vi "Linear Fit (single).vi"(8 "error in (no error)":errorcluster, 9 "Type":enum16{"y vs x", "x vs y"}(ring), 11 "XY-data":cluster{"X-array":dbl[], "Y-array":dbl[]}) -> (0 "error out":errorcluster, 2 "Best Fit":cluster{"X-array":dbl[], "Y-array":dbl[]} {"Y-array" format="%.2p"; "X-array" format="%.2p"}, 3 "XY-data out":cluster{"X-array":dbl[], "Y-array":dbl[]}, 4 "slope":dbl, 5 "Lower Bound":cluster{"X-array":dbl[], "Y-array":dbl[]}, 6 "intercept":dbl, 7 "Upper Bound":cluster{"X-array":dbl[], "Y-array":dbl[]})   [LabVIEW 2019, in "xy_utilities.lvlib"]
doc: "Performs a linear fit using linear LS algorithm.\n\nWire data to the data input to determine the polymorphic instance to use or manually select the instance."
uses:
  xy_utilities.lvlib
  <vilib>/Analysis/6fits.llb/Curve Fitting Criteria.ctl
  Swap X and Y (single).vi
  <vilib>/Analysis/6fits.llb/Confidence Interval (Linear).vi
  <vilib>/Analysis/NI_AALPro.lvlib
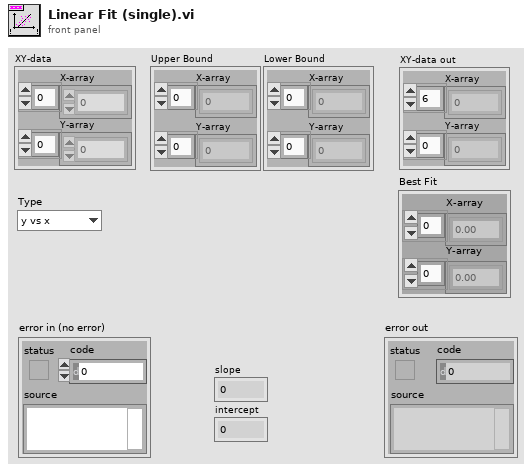
[diagram p1: front panel]
types:
  T1 = typedef "NI_AALPro.lvlib/Curve Fitting Criteria.ctl" = u16
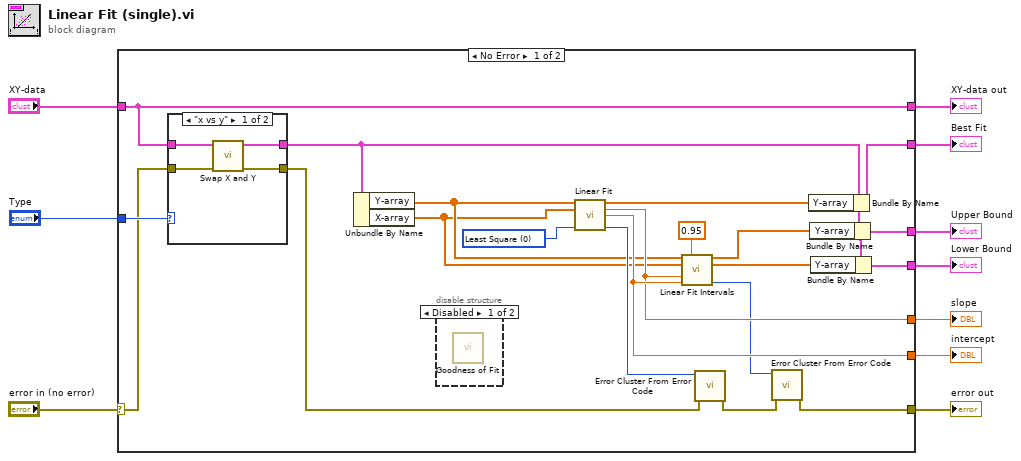
[diagram p0: block diagram]
diagram:
  n1 = case shown="No Error" "error in (no error)" {
    selector: "error in (no error)" -> [w30 w39]
    tunnel: [w18 w39] -> w9
    tunnel: "XY-data" -> [w28 w38]
    tunnel: [w29 _] -> w7
    tunnel: "Type" -> [w31 _]
    tunnel: [w28 w38] -> w5
    tunnel: [w22 _] -> w4
    tunnel: [w23 _] -> w3
    tunnel: [w12 _] -> w2
    tunnel: [w11 _] -> w1
    frame No Error {
      w24 = T1 0 items=["Least Square", "Least Absolute Residual", "Bisquare"] ("method")
      n2 = case shown="\"x vs y\"" w31 {
        tunnel: w28 -> [w35 w37]
        tunnel: [w34 w37] -> w13
        tunnel: [w33 w36] -> w27
        tunnel: w30 -> [w32 w36]
        frame "x vs y" {
          n3 = call-poly "Swap X and Y.vi"("error in (no error)"=w32, "XY-data"=w35) -> ("error out"=w33:errorcluster, "XY-data out"=w34:cluster{"X-array":dbl[], "Y-array":dbl[]})  [unwired: 8 in]
        }
        frame "y vs x" {
        }
      }
      n4 = Unbundle By Name(w13) -> ("Y-array"=w17:dbl[], "X-array"=w16:dbl[])
      n5 = disable-structure shown="Disabled" {
        frame Disabled {
          n6 = call <vilib>:"Goodness of Fit.vi"() -> ()  [unwired: 8 in, 4 out]
        }
        frame Enabled {
        }
      }
      n7 = call <vilib>:"Linear Fit.vi"("Y"=w17, "X"=w16, "method"=w24) -> ("Best Linear Fit"=w26:dbl[], "slope"=w22:dbl, "intercept"=w23:dbl, "error"=w25:i32)  [unwired: 8 in, 1 out]
      n8 = call-poly <vilib>:"Linear Fit Intervals.vi"("Y"=w17, "confidence level"=0.95, "X"=w16, "slope"=w22, "intercept"=w23) -> ("Upper Bound"=w15:dbl[], "Lower Bound"=w14:dbl[], "error"=w20:i32)  [unwired: 6 in, 2 out]
      n9 = call <vilib>:"Error Cluster From Error Code.vi"("error in (no error)"=w27, "error code (0)"=w25) -> ("error out"=w19:errorcluster)  [unwired: 7 in]
      n10 = call <vilib>:"Error Cluster From Error Code.vi"("error in (no error)"=w19, "error code (0)"=w20) -> ("error out"=w18:errorcluster)  [unwired: 7 in]
      n11 = Bundle By Name(cluster=w13, "Y-array"=w26) -> (w29:cluster{"X-array":dbl[], "Y-array":dbl[]})
      n12 = Bundle By Name(cluster=w13, "Y-array"=w15) -> (w12:cluster{"X-array":dbl[], "Y-array":dbl[]})
      n13 = Bundle By Name(cluster=w13, "Y-array"=w14) -> (w11:cluster{"X-array":dbl[], "Y-array":dbl[]})
    }
    frame Error {
    }
  }
  "error out" <- w9
  "Best Fit" <- w7
  "XY-data out" <- w5
  "slope" <- w4
  "intercept" <- w3
  "Upper Bound" <- w2
  "Lower Bound" <- w1
